vi "SEND KEVIN EMAILS.vi"(9 "DAYS BETWEEN REMINDERS":string="3", 10 "DAYS BEFORE DUE DATE":string="1", 11 "connection reference in":T1) -> (3 "connection reference out":T1)   [LabVIEW 2019]
uses:
  <vilib>/addons/database/Connection.llb/Conn ObjectReference.ctl
  <vilib>/addons/database/Auxilliary.llb/DB Tools Cursor Type.ctl
  <vilib>/addons/database/Connection.llb/Conn Execute.vi
  <vilib>/addons/database/Recordset.llb/Rec Fetch Recordset Data (R).vi
  <vilib>/addons/database/Recordset.llb/Rec Destroy - Connection.vi
  <vilib>/addons/database/_DB Variant To Data/Database Variant To Data.xnode
  <vilib>/addons/database/NI_Database_API.lvlib
panel:
  out "Emails":string[](array[string])
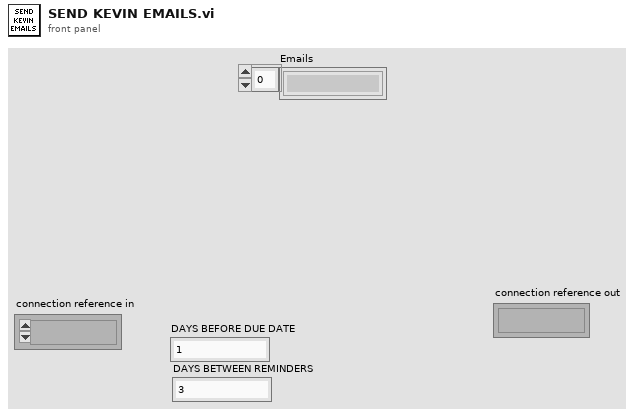
[diagram p1: front panel]
types:
  T1 = typedef "NI_Database_API.lvlib/Conn ObjectReference.ctl" = refnum<k1>
  T2 = typedef "NI_Database_API.lvlib/DB Tools Cursor Type.ctl" = enum16{"forward-only", "keyset", "dynamic", "static"}
  T3 = typedef "LVDateTimeRec.ctl" = cluster{"fractional second":dbl, "second":i32, "minute":i32, "hour":i32, "day of month":i32, "month":i32, "year":i32, "day of week":i32, "day of year":i32, "DST":i32}
  T4 = typedef "NI_Database_API.lvlib/Rec ObjectReference.ctl" = refnum<k1>
  T5 = typedef "Inventory Data Type.ctl" = cluster{"Identifier":string, "BYU ICN #":string, "Item Description":string, "Comments":string, "Checked Out Date":string, "Due Date":string, "Check Out Location":string, "Reminder Count":i32, "Most Recent Reminder Date":string, "BYU ID #":string, "Building/Room":string, "Location in Room":string, "Manual":string, "Manufacturer":string, "Model #":string, "Serial #":string, "Date Acquired":string, "Reminder Notes":string}
  T6 = cluster{"NOT DUE ITEMS":T5[], "DUE ITEMS":T5[], "REMINDER ITEMS":T5[], "EARLY REMINDER ITEMS":T5[]}
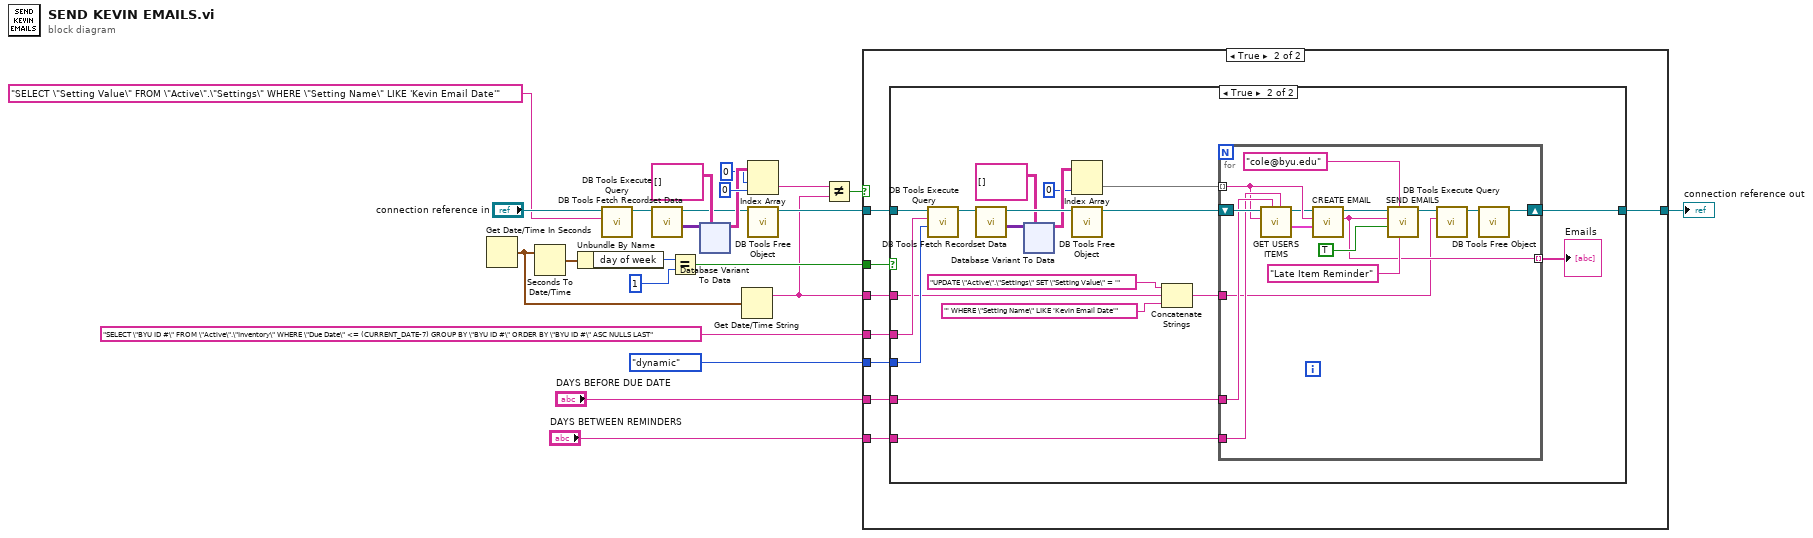
[diagram p0: block diagram]
diagram:
  n1 = Get Date/Time In Seconds() -> (seconds since 1Jan1904=w12:timestamp)
  n2 = Seconds To Date/Time(time stamp (now)=w12) -> (date time rec=w23:T3)  [unwired: 1 in]
  n3 = Unbundle By Name(w23) -> ("day of week"=w22:i32)
  n4 = call-poly <vilib>:"DB Tools Execute Query.vi"("SQL query"="SELECT \"Setting Value\" FROM \"Active\".\"Settings\" WHERE \"Setting Name\" LIKE 'Kevin Email Date'", "connection reference"="connection reference in") -> ("recordset reference"=w6:T4)  [unwired: 6 in, 1 out]
  n5 = call-poly <vilib>:"DB Tools Fetch Recordset Data.vi"("recordset reference"=w6) -> ("recordset data"=w9:variant[][], "recordset reference out"=w7:T4)  [unwired: 4 in, 1 out]
  n6 = Equal?(x=w22, y=1) -> (x = y?=w20:bool)
  n7 = xnode "Database Variant To Data"("database variant"=w9, "type"=string[][] []) -> ("data"=w8:string[][])  [unwired: 1 in, 1 out]
  n8 = Get Date/Time String(seconds (now)=w12) -> (date string=w1:string)  [unwired: 2 in, 1 out]
  n9 = Index Array(array=w8, index (row)=0 ("disabled index (row)"), index (col)=0 ("disabled index (col)")) -> (element=w3:string)
  n10 = call-poly <vilib>:"DB Tools Free Object.vi"("recordset reference"=w7) -> ("connection reference"=w5:T1)  [unwired: 9 in, 1 out]
  n11 = Not Equal?(x=w3, y=w1) -> (x != y?=w2:bool)
  n12 = case shown="True" w2 {
    tunnel: w20 -> [_ w32]
    tunnel: w5 -> [w24 w31]
    tunnel: [w24 w30] -> w19
    tunnel: "SELECT \"BYU ID #\" FROM \"Active\".\"Inventory\" WHERE \"Due Date\" <= (CURRENT_DATE-7) GROUP BY \"BYU ID #\" ORDER BY \"BYU ID #\" ASC NULLS LAST" -> [_ w29]
    tunnel: DB_Tools_Cursor_Type."dynamic" ("cursor type") -> [_ w28]
    tunnel: "DAYS BEFORE DUE DATE" -> [_ w27]
    tunnel: "DAYS BETWEEN REMINDERS" -> [_ w26]
    tunnel: w1 -> [_ w25]
    frame False {
    }
    frame True {
      n13 = case shown="True" w32 {
        tunnel: w31 -> [w33 w46]
        tunnel: [w33 w39] -> w30
        tunnel: w29 -> [_ w45]
        tunnel: w28 -> [_ w44]
        tunnel: w27 -> [_ w41]
        tunnel: w26 -> [_ w40]
        tunnel: w25 -> [_ w36]
        frame False {
        }
        frame True {
          n14 = call-poly <vilib>:"DB Tools Execute Query.vi"("cursor type"=w44, "SQL query"=w45, "connection reference"=w46) -> ("recordset reference"=w49:T4)  [unwired: 5 in, 1 out]
          n15 = call-poly <vilib>:"DB Tools Fetch Recordset Data.vi"("recordset reference"=w49) -> ("recordset data"=w50:variant[][], "recordset reference out"=w52:T4)  [unwired: 4 in, 1 out]
          n16 = xnode "Database Variant To Data"("database variant"=w50, "type"=string[][] []) -> ("data"=w51:string[][])  [unwired: 1 in, 1 out]
          n17 = Index Array(array=w51, index (col)=0 ("disabled index (col)")) -> (element=w43:string[])  [unwired: 1 in]
          n18 = call-poly <vilib>:"DB Tools Free Object.vi"("recordset reference"=w52) -> ("connection reference"=w42:T1)  [unwired: 9 in, 1 out]
          n19 = Concatenate Strings("UPDATE \"Active\".\"Settings\" SET \"Setting Value\" = '" ("SQL query"), w36, "' WHERE \"Setting Name\" LIKE 'Kevin Email Date'" ("string")) -> (w34:string)
          n20 = for {
            tunnel: w43 -> [w64] mode=indexing
            shift-right: [w53] -> w39
            shift-left: w42 -> [w67]
            tunnel: w41 -> [w66]
            tunnel: w40 -> [w65]
            tunnel: [w57] -> w38 mode=indexing
            tunnel: w34 -> [w55]
            n21 = call "GET USERS ITEMS.vi"("DAYS BETWEEN REMINDERS"=w65, "DAYS BEFORE DUE DATE"=w66, "BYU ID # IN"=w64, "connection reference in"=w67) -> ("DATA OUT"=w62:T6, "connection reference out"=w63:T1)  [unwired: 6 in]
            n22 = call "CREATE EMAIL.vi"("DATA IN"=w62, "BYU ID # IN"=w64, "connection reference in"=w63) -> ("MESSAGE OUT"=w57:string, "connection reference out"=w61:T1)  [unwired: 4 in, 3 out]
            n23 = call "SEND EMAILS.vi"("Subject"="Late Item Reminder", "USER EMAIL IN"="cole@byu.edu", "SEND EMAIL"=TRUE, "MESSAGE IN"=w57, "connection reference in"=w61) -> ("connection reference out"=w56:T1)  [unwired: 6 in]
            n24 = call-poly <vilib>:"DB Tools Execute Query.vi"("SQL query"=w55, "connection reference"=w56) -> ("recordset reference"=w54:T4)  [unwired: 6 in, 1 out]
            n25 = call-poly <vilib>:"DB Tools Free Object.vi"("recordset reference"=w54) -> ("connection reference"=w53:T1)  [unwired: 9 in, 1 out]
          }
          "Emails" <- w38
        }
      }
    }
  }
  "connection reference out" <- w19
